vi "Lines Filter-[].vi"(8 "error in (no error)":errorcluster, 11 "Lines":string[](array[string])) -> (0 "error out":errorcluster, 3 "Config Text List":string[](array[string]))   [LabVIEW 2012]
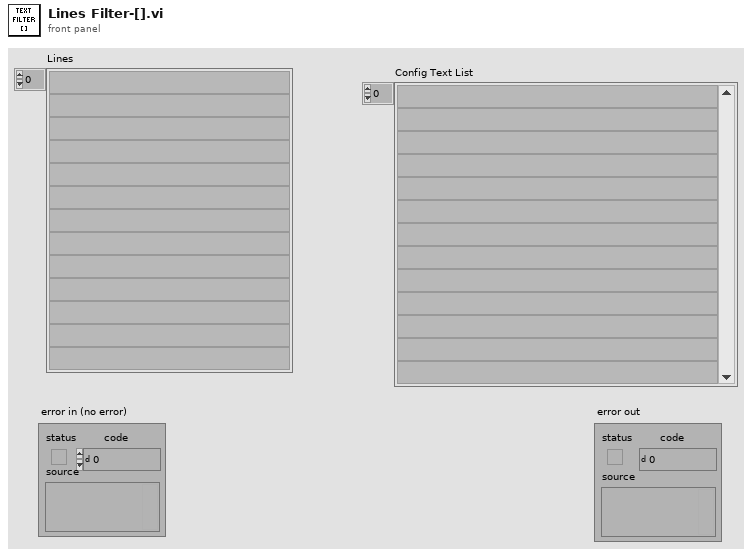
[diagram p1: front panel]
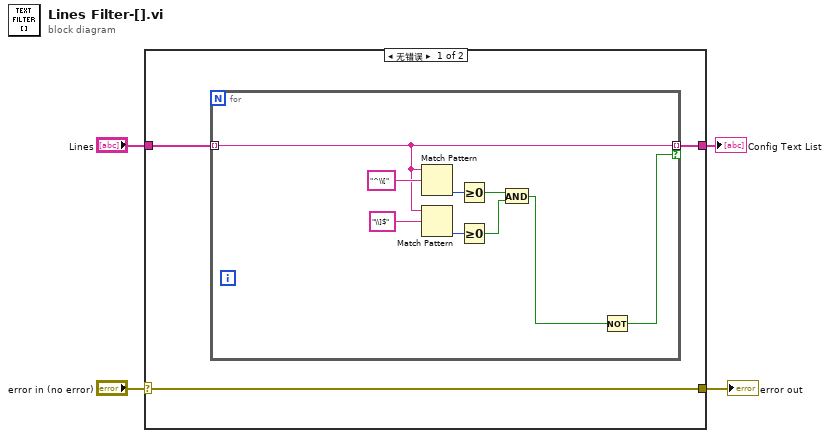
[diagram p0: block diagram]
diagram:
  n1 = case shown="无错误" "error in (no error)" {
    selector: "error in (no error)" -> [w5 w17]
    tunnel: [w5 w17] -> w3
    tunnel: "Lines" -> [w7 _]
    tunnel: [w6 _] -> w1
    frame No Error {
      n2 = for {
        tunnel: w7 -> [w8] mode=indexing
        tunnel: [w8] -> w6 mode=indexing if=w9
        n3 = Match Pattern(string=w8, regular expression="^\\[") -> (offset past match=w15:i32)  [unwired: 1 in, 3 out]
        n4 = Match Pattern(string=w8, regular expression="\\]$") -> (offset past match=w14:i32)  [unwired: 1 in, 3 out]
        n5 = Greater Or Equal To 0?(x=w15) -> (x >= 0?=w12:bool)
        n6 = Greater Or Equal To 0?(x=w14) -> (x >= 0?=w11:bool)
        n7 = And(x=w12, y=w11) -> (x .and. y?=w10:bool)
        n8 = Not(x=w10) -> (.not. x?=w9:bool)
      }
    }
    frame Error {
    }
  }
  "error out" <- w3
  "Config Text List" <- w1
